vi "aula2.vi"() -> ()   [LabVIEW 2020]
panel:
  in  "Boolean":bool
  out "ºC":dbl(slide) scale=0.0..100.0
  in  "ºF":dbl(slide) scale=0.0..10.0
  in  "milliseconds to wait":u32
  out "Indicador":i32
  in  "Stop":bool
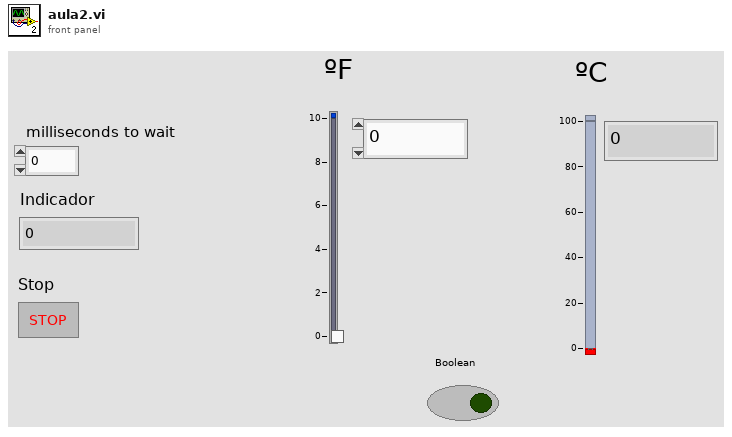
[diagram p1: front panel]
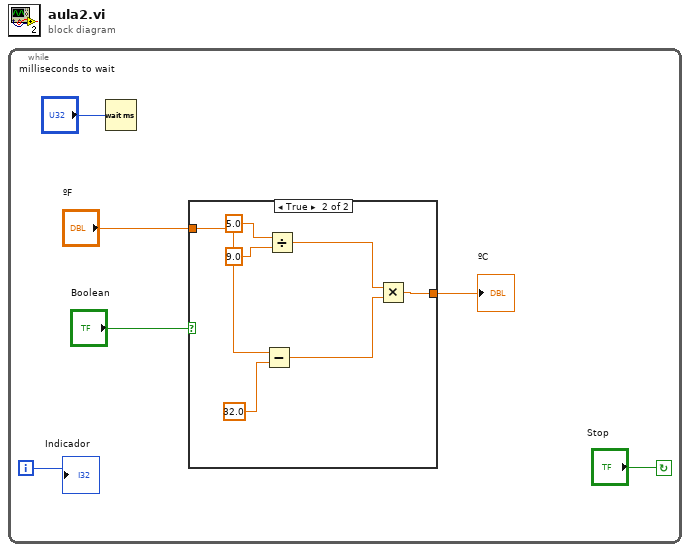
[diagram p0: block diagram]
diagram:
  n1 = while {
    i -> [w5]
    stop <- "Stop" continue-if-true
    n2 = Wait (ms)(milliseconds to wait="milliseconds to wait") -> ()  [unwired: 1 out]
    n3 = case shown="True" "Boolean" {
      tunnel: "ºF" -> [w7 w12]
      tunnel: [w7 w8] -> w2
      frame False {
      }
      frame True {
        n4 = Subtract(x=w12, y=32.0) -> (x-y=w9:dbl)
        n5 = Divide(x=5.0, y=9.0) -> (x/y=w10:dbl)
        n6 = Multiply(x=w10, y=w9) -> (x*y=w8:dbl)
      }
    }
    "ºC" <- w2
    "Indicador" <- w5
  }
